vi "Tree.vi"   [LabVIEW 2021]
panel:
  # "SSI OE1022D库函数"
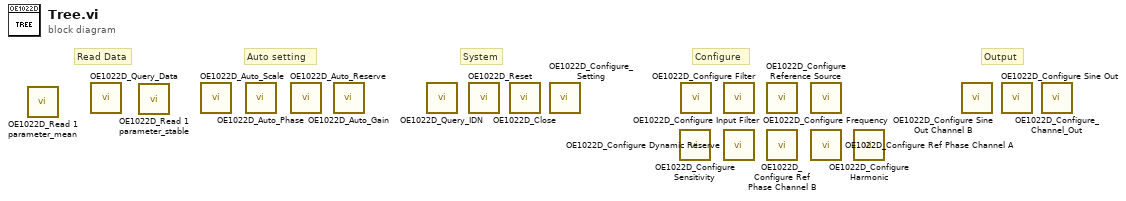
[diagram p0: block diagram]
diagram:
  # "Output"
  # "Configure"
  # "System"
  # "Read Data"
  # "Auto setting"
  n1 = call <instrlib>:"OE1022D_Read 1 parameter_mean.vi"() -> ()  [unwired: 9 in, 3 out]
  n2 = call <instrlib>:"OE1022D_Query_Data.vi"() -> ()  [unwired: 5 in, 5 out]
  n3 = call <instrlib>:"OE1022D_Read 1 parameter_stable.vi"() -> ()  [unwired: 9 in, 3 out]
  n4 = call <instrlib>:"OE1022D_Auto_Scale.vi"() -> ()  [unwired: 18 in, 2 out]
  n5 = call <instrlib>:"OE1022D_Auto_Phase.vi"() -> ()  [unwired: 18 in, 2 out]
  n6 = call <instrlib>:"OE1022D_Auto_Reserve.vi"() -> ()  [unwired: 18 in, 2 out]
  n7 = call <instrlib>:"OE1022D_Auto_Gain.vi"() -> ()  [unwired: 18 in, 2 out]
  n8 = call <instrlib>:"OE1022D_Query_IDN.vi"() -> ()  [unwired: 3 in, 3 out]
  n9 = call <instrlib>:"OE1022D_Reset.vi"() -> ()  [unwired: 18 in, 2 out]
  n10 = call <instrlib>:"OE1022D_Close.vi"() -> ()  [unwired: 3 in, 1 out]
  n11 = call <instrlib>:"OE1022D_Configure_Setting.vi"() -> ()  [unwired: 5 in, 2 out]
  n12 = call <instrlib>:"OE1022D_Configure Sensitivity.vi"() -> ()  [unwired: 18 in, 2 out]
  n13 = call <instrlib>:"OE1022D_Configure Input Filter.vi"() -> ()  [unwired: 14 in, 2 out]
  n14 = call <instrlib>:"OE1022D_Configure Filter.vi"() -> ()  [unwired: 10 in, 2 out]
  n15 = call <instrlib>:"OE1022D_Configure Dynamic Reserve.vi"() -> ()  [unwired: 17 in, 3 out]
  n16 = call <instrlib>:"OE1022D_Configure Reference Source.vi"() -> ()  [unwired: 18 in, 2 out]
  n17 = call <instrlib>:"OE1022D_Configure Ref Phase Channel B.vi"() -> ()  [unwired: 18 in, 2 out]
  n18 = call <instrlib>:"OE1022D_Configure Frequency.vi"() -> ()  [unwired: 18 in, 2 out]
  n19 = call <instrlib>:"OE1022D_Configure Ref Phase Channel A.vi"() -> ()  [unwired: 18 in, 2 out]
  n20 = call <instrlib>:"OE1022D_Configure Harmonic.vi"() -> ()  [unwired: 18 in, 2 out]
  n21 = call <instrlib>:"OE1022D_Configure Sine Out Channel B.vi"() -> ()  [unwired: 14 in, 2 out]
  n22 = call <instrlib>:"OE1022D_Configure Sine Out.vi"() -> ()  [unwired: 14 in, 2 out]
  n23 = call <instrlib>:"OE1022D_Configure_Channel_Out.vi"() -> ()  [unwired: 14 in, 2 out]
